vi "save B scan data in binary.vi"(10 "Channel array in":sgl[][](array[numeric]), 11 "Scan save path":path) -> (3 "Size":i32[](array[numeric]))   [LabVIEW 2014]
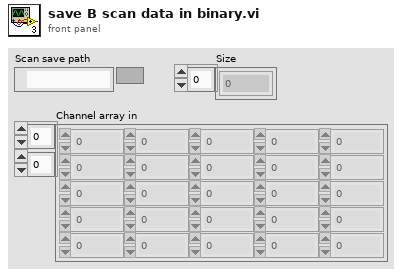
[diagram p1: front panel]
types:
  T1 = enum16{"open", "replace", "create", "open or create", "replace or create", "replace or create with confirmation"}
  T2 = enum16{"big-endian, network order", "native, host order", "little-endian"}
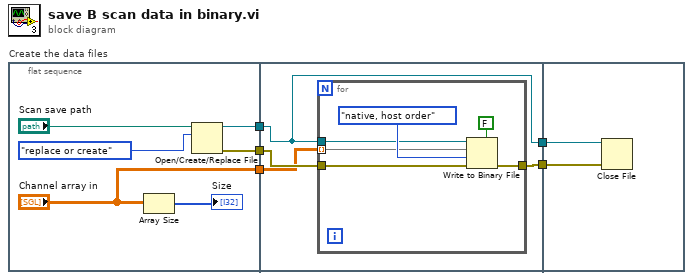
[diagram p0: block diagram]
diagram:
  n1 = flat-sequence "Create the data files" {
    tunnel: [w10] -> w5
    tunnel: ["Channel array in"] -> w4
    tunnel: [w6] -> w3
    tunnel: w5 -> [w15]
    tunnel: w4 -> [w14]
    tunnel: w3 -> [w12]
    tunnel: [w12] -> w2
    tunnel: [w13] -> w1
    tunnel: w2 -> [w23]
    tunnel: w1 -> [w22]
    frame #0 {
      n2 = Array Size(array="Channel array in") -> (size(s)=→"Size":i32[])
      n3 = Open/Create/Replace File(file path (use dialog)="Scan save path", operation (0:open)=T1."replace or create") -> (refnum out=w6:refnum<file>, error out=w10:errorcluster)  [unwired: 4 in, 1 out]
    }
    frame #1 {
      n4 = for {
        tunnel: [w20] -> w13
        tunnel: w12 -> [w18]
        tunnel: w15 -> [w17]
        tunnel: w14 -> [w16] mode=indexing
        n5 = Write to Binary File(file (use dialog)=w18, data=w16, error in=w17, 5:FALSE ("prepend array or string size? (T)"), 9:T2."native, host order" ("byte order (0:big-endian, network order)")) -> (error out=w20:errorcluster)  [unwired: 1 in, 2 out]
      }
    }
    frame #2 {
      n6 = Close File(refnum=w23, error in=w22) -> ()  [unwired: 2 out]
    }
  }
